vi "sequence2pb_commands.vi"(4 "Refocus_s":u32, 6 "Repetitions":i32, 7 "Refocus?":bool, 9 "command_sequence":T1(array[cluster]), 10 "Sequence_length":dbl, 11 "start_command":i32) -> (1 "end_command":i32, 2 "t_remaining":dbl format="%#_13g", 3 "PB_commands":T1(array[cluster]))   [LabVIEW 2018]
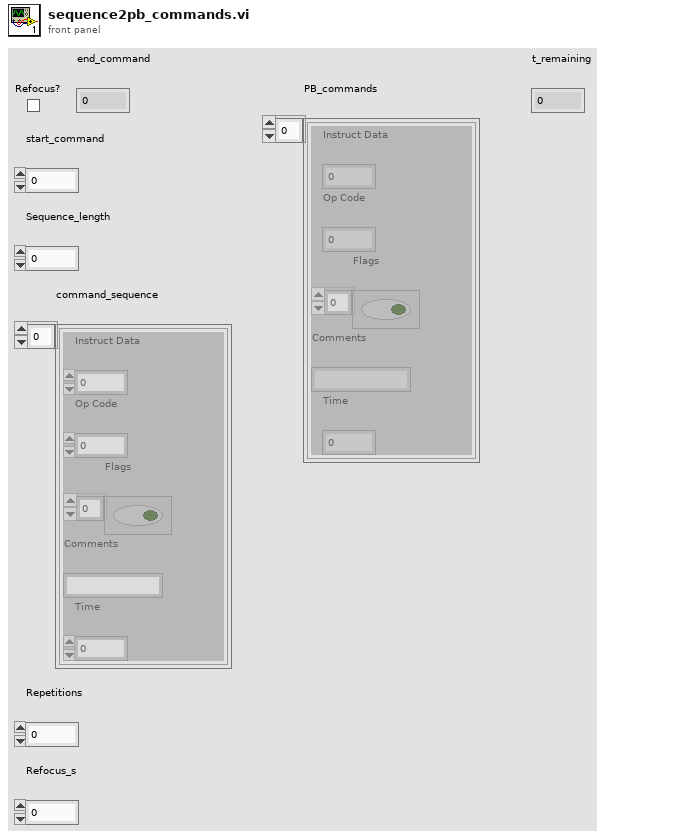
[diagram p1: front panel]
types:
  T1 = cluster{"Instruct Data":i32, "Op Code":i32, "Flags":bool[], "Comments":string, "Time":dbl}[]
  T2 = cluster{"Instruct Data":i32, "Op Code":i32, "Flags":bool[], "Comments":string, "Time":dbl}
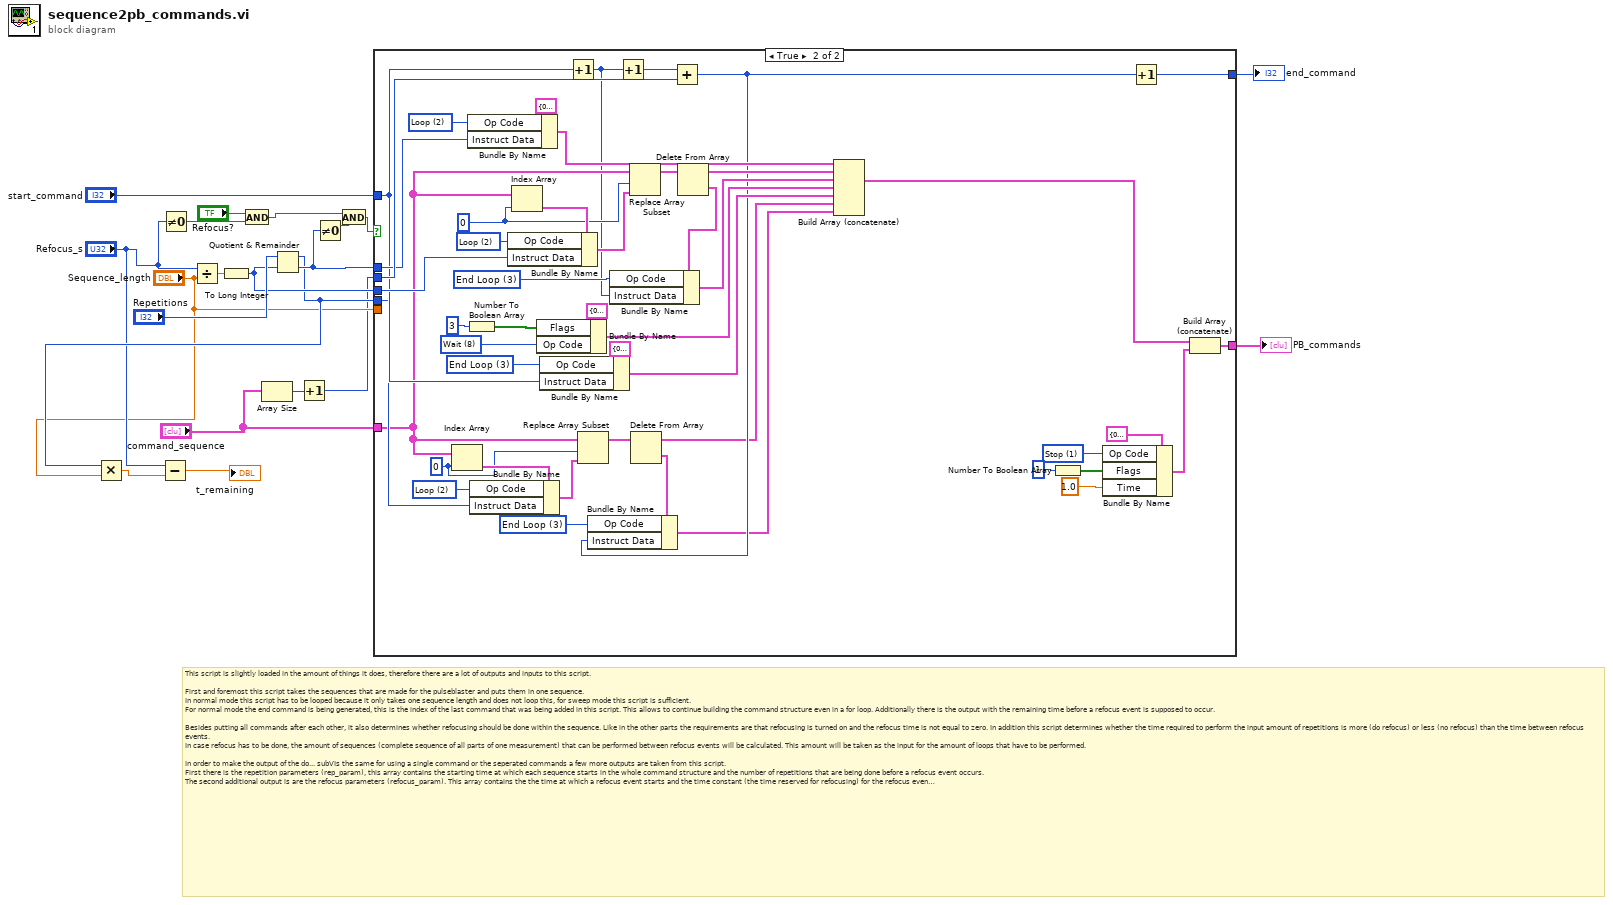
[diagram p0: block diagram]
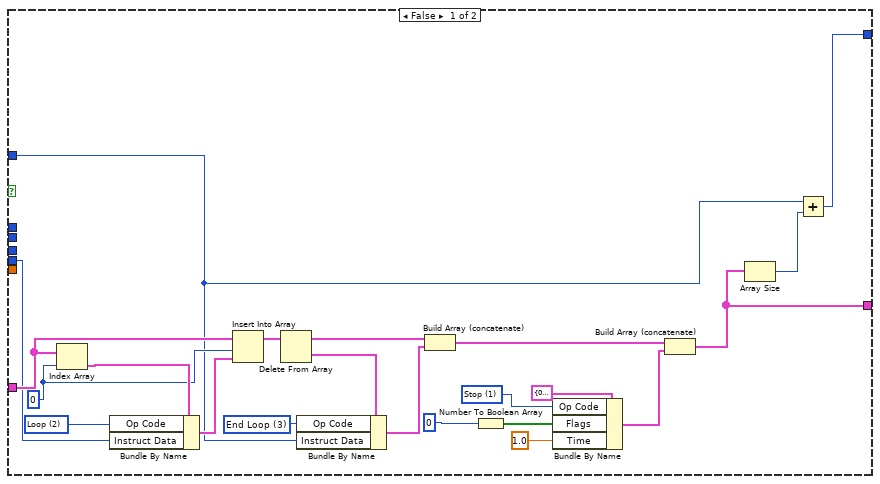
[diagram p2: hidden frame]
diagram:
  # "This script is slightly loaded in the amount of things it does, therefore there are a lot of outputs and inputs to this script.\n\nFirst and foremost this script takes the sequences that are made for the pulseblaster and puts them in one sequence. \nIn normal mode this script has to be looped because it only takes one sequence length and does not loop this, for sweep mode this script is sufficient.\nFor normal mode the end command is being generated, this is the index of the last command that was being added in this script. This allows to continue building the command structure even in a for loop. Additionally there is the output with the remaining time before a refocus event is supposed to occur.\n\nBesides putting all commands after each other, it also determines whether refocusing should be done within the sequence. Like in the other parts the requirements are that refocusing is turned on and the refocus time is not equal to zero. In addition this script determines whether the time required to perform the input amount of repetitions is more (do refocus) or less (no refocus) than the time between refocus events.\nIn case refocus has to be done, the amount of sequences (complete sequence of all parts of one measurement) that can be performed between refocus events will be calculated. This amount will be taken as the input for the amount of loops that have to be performed.\n\nIn order to make the output of the do... subVIs the same for using a single command or the seperated commands a few more outputs are taken from this script. \nFirst there is the repetition parameters (rep_param), this array contains the starting time at which each sequence starts in the whole command structure and the number of repetitions that are being done before a refocus event occurs.\nThe second additional output is are the refocus parameters (refocus_param). This array contains the the time at which a refocus event starts and the time constant (the time reserved for refocusing) for the refocus event."
  n1 = Not Equal To 0?(x="Refocus_s") -> (x != 0?=w15:bool)
  n2 = Divide(x="Refocus_s", y="Sequence_length") -> (x/y=w12:dbl)
  n3 = To Long Integer(number=w12) -> (32bit integer=w7:i32)
  n4 = And(x="Refocus?", y=w15) -> (x .and. y?=w17:bool)
  n5 = Array Size(array="command_sequence") -> (size(s)=w14:i32)
  n6 = Quotient & Remainder(x="Repetitions", y=w7) -> (x-y*floor(x/y)=w5:i32, floor(x/y)=w6:i32)
  n7 = Multiply(x=w5, y="Sequence_length") -> (x*y=w9:dbl)
  n8 = Subtract(x="Refocus_s", y=w9) -> (x-y=→"t_remaining":dbl)
  n9 = Increment(x=w14) -> (x+1=w1:i32)
  n10 = Not Equal To 0?(x=w6) -> (x != 0?=w20:bool)
  n11 = And(x=w17, y=w20) -> (x .and. y?=w18:bool)
  n12 = case shown="True" w18 {
    tunnel: w7 -> [_ w61]
    tunnel: [w25 w82] -> w19
    tunnel: "command_sequence" -> [w40 w53]
    tunnel: w1 -> [_ w89]
    tunnel: w6 -> [_ w63]
    tunnel: w5 -> [w21 w54]
    tunnel: [w23 w81] -> w11
    tunnel: "start_command" -> [w22 w58]
    tunnel: "Sequence_length" -> [_ _]
    frame False {
      w31 = 1 items=["Continue", "Stop", "Loop", "End Loop", "JSR", "RTS", "Branch", "Long Delay", "Wait"] ("Op Code 2")
      w36 = 3 items=["Continue", "Stop", "Loop", "End Loop", "JSR", "RTS", "Branch", "Long Delay", "Wait"] ("Op Code 2")
      w41 = 2 items=["Continue", "Stop", "Loop", "End Loop", "JSR", "RTS", "Branch", "Long Delay", "Wait"] ("Op Code 2")
      w35 = 0
      n13 = Index Array(array=w40, index=w35) -> (element=w42:T2)
      n14 = Bundle By Name(cluster=w42, "Op Code"=w41, "Instruct Data"=w21) -> (w39:T2)
      n15 = Insert Into Array(array=w40, index=w35, new element=w39) -> (w38:T1)
      n16 = Delete From Array(array=w38) -> (deleted portion=w37:T2, array with subset deleted=w33:T1)  [unwired: 2 in]
      n17 = Bundle By Name(cluster=w37, "Op Code"=w36, "Instruct Data"=w22) -> (w34:T2)
      n18 = Build Array (concatenate)(w33, w34) -> (w27:T1)
      n19 = Number To Boolean Array(number=0) -> (Boolean array=w29:bool[])
      n20 = Bundle By Name(cluster=T2 {"Instruct Data"=0, "Op Code"=0, "Flags"=[FALSE, FALSE, FALSE, FALSE, FALSE, FALSE, FALSE, FALSE, FALSE, FALSE, FALSE, FALSE, FALSE, FALSE, FALSE, FALSE, FALSE, FALSE, FALSE, FALSE, FALSE, FALSE, FALSE, FALSE], "Comments"="", "Time"=1e-06} ("PB Instruction"), "Op Code"=w31, "Flags"=w29, "Time"=1.0) -> (w26:T2)
      n21 = Build Array (concatenate)(w27, w26) -> (w25:T1)
      n22 = Array Size(array=w25) -> (size(s)=w24:i32)
      n23 = Add(x=w22, y=w24) -> (x+y=w23:i32)
    }
    frame True {
      w48 = 3 items=["Continue", "Stop", "Loop", "End Loop", "JSR", "RTS", "Branch", "Long Delay", "Wait"] ("Op Code 2")
      w55 = 2 items=["Continue", "Stop", "Loop", "End Loop", "JSR", "RTS", "Branch", "Long Delay", "Wait"] ("Op Code 2")
      w52 = 0 ("index")
      w59 = 3 items=["Continue", "Stop", "Loop", "End Loop", "JSR", "RTS", "Branch", "Long Delay", "Wait"] ("Op Code 2")
      w64 = 2 items=["Continue", "Stop", "Loop", "End Loop", "JSR", "RTS", "Branch", "Long Delay", "Wait"] ("Op Code 2")
      w67 = 8 items=["Continue", "Stop", "Loop", "End Loop", "JSR", "RTS", "Branch", "Long Delay", "Wait"] ("Op Code 2")
      w74 = 0
      w73 = 3 items=["Continue", "Stop", "Loop", "End Loop", "JSR", "RTS", "Branch", "Long Delay", "Wait"] ("Op Code 2")
      w77 = 2 items=["Continue", "Stop", "Loop", "End Loop", "JSR", "RTS", "Branch", "Long Delay", "Wait"] ("Op Code 2")
      w88 = 1 items=["Continue", "Stop", "Loop", "End Loop", "JSR", "RTS", "Branch", "Long Delay", "Wait"] ("Op Code 2")
      n24 = Index Array(array=w53, index=w52) -> (element=w56:T2)
      n25 = Number To Boolean Array(number=3) -> (Boolean array=w69:bool[])
      n26 = Bundle By Name(cluster=T2 {"Instruct Data"=0, "Op Code"=0, "Flags"=[FALSE, FALSE, FALSE, FALSE, FALSE, FALSE, FALSE, FALSE, FALSE, FALSE, FALSE, FALSE, FALSE, FALSE, FALSE, FALSE, FALSE, FALSE, FALSE, FALSE, FALSE, FALSE, FALSE, FALSE], "Comments"="", "Time"=1e-06} ("PB Instruction"), "Op Code"=w64, "Instruct Data"=w63) -> (w62:T2)
      n27 = Bundle By Name(cluster=w56, "Op Code"=w55, "Instruct Data"=w54) -> (w51:T2)
      n28 = Index Array(array=w53, index=w74) -> (element=w76:T2)
      n29 = Bundle By Name(cluster=w76, "Op Code"=w77, "Instruct Data"=w61) -> (w75:T2)
      n30 = Bundle By Name(cluster=T2 {"Instruct Data"=0, "Op Code"=0, "Flags"=[FALSE, FALSE, FALSE, FALSE, FALSE, FALSE, FALSE, FALSE, FALSE, FALSE, FALSE, FALSE, FALSE, FALSE, FALSE, FALSE, FALSE, FALSE, FALSE, FALSE, FALSE, FALSE, FALSE, FALSE], "Comments"="", "Time"=1e-06} ("PB Instruction"), "Flags"=w69, "Op Code"=w67) -> (w66:T2)
      n31 = Bundle By Name(cluster=T2 {"Instruct Data"=0, "Op Code"=0, "Flags"=[FALSE, FALSE, FALSE, FALSE, FALSE, FALSE, FALSE, FALSE, FALSE, FALSE, FALSE, FALSE, FALSE, FALSE, FALSE, FALSE, FALSE, FALSE, FALSE, FALSE, FALSE, FALSE, FALSE, FALSE], "Comments"="", "Time"=1e-06} ("PB Instruction"), "Op Code"=w59, "Instruct Data"=w58) -> (w57:T2)
      n32 = Increment(x=w58) -> (x+1=w43:i32)
      n33 = Replace Array Subset(array=w53, new element=w51, index=w52) -> (w50:T1)
      n34 = Increment(x=w43) -> (x+1=w44:i32)
      n35 = Replace Array Subset(array=w53, new element=w75, index=w74) -> (w79:T1)
      n36 = Delete From Array(array=w50) -> (deleted portion=w49:T2, array with subset deleted=w46:T1)  [unwired: 2 in]
      n37 = Add(x=w44, y=w89) -> (x+y=w47:i32)
      n38 = Bundle By Name(cluster=w49, "Op Code"=w48, "Instruct Data"=w47) -> (w45:T2)
      n39 = Delete From Array(array=w79) -> (deleted portion=w68:T2, array with subset deleted=w72:T1)  [unwired: 2 in]
      n40 = Bundle By Name(cluster=w68, "Op Code"=w73, "Instruct Data"=w43) -> (w71:T2)
      n41 = Build Array (concatenate)(w62, w72, w71, w66, w57, w46, w45) -> (w84:T1)
      n42 = Number To Boolean Array(number=1) -> (Boolean array=w86:bool[])
      n43 = Bundle By Name(cluster=T2 {"Instruct Data"=0, "Op Code"=0, "Flags"=[FALSE, FALSE, FALSE, FALSE, FALSE, FALSE, FALSE, FALSE, FALSE, FALSE, FALSE, FALSE, FALSE, FALSE, FALSE, FALSE, FALSE, FALSE, FALSE, FALSE, FALSE, FALSE, FALSE, FALSE], "Comments"="", "Time"=1e-06} ("PB Instruction"), "Op Code"=w88, "Flags"=w86, "Time"=1.0) -> (w83:T2)
      n44 = Increment(x=w47) -> (x+1=w81:i32)
      n45 = Build Array (concatenate)(w84, w83) -> (w82:T1)
    }
  }
  "PB_commands" <- w19
  "end_command" <- w11
